vi "DSF.Shared.Configuration.Framework.Collapse Cluster.vi"(8 "error in (no error)":errorcluster, 11 "Framework Configuration in":refnum<class "DSF.Shared.Configuration.Framework.lvclass">) -> (0 "error out":errorcluster, 3 "Framework Configuration out":refnum<class "DSF.Shared.Configuration.Framework.lvclass">)   [LabVIEW 2017, in "DSF.Engine.lvlib" / "DSF.Shared.Configuration.Framework.lvclass"]
uses:
  DSF.Shared.Configuration.Framework.lvclass
  DSF.Shared.Configuration.Framework.lvclass/DSF.Shared.Configuration.Framework.ctl
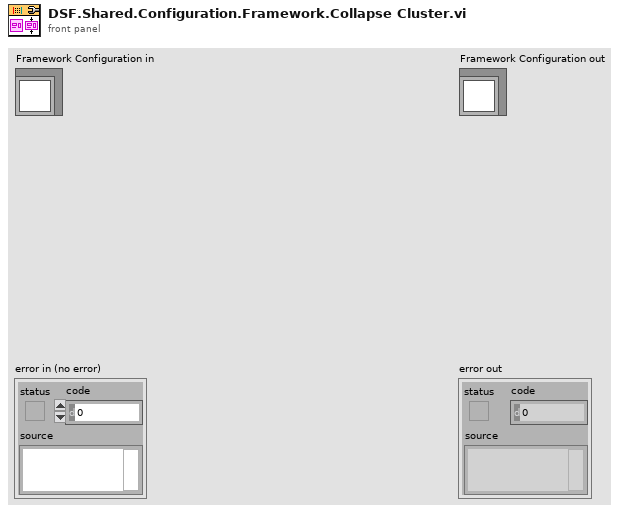
[diagram p1: front panel]
types:
  T1 = typedef "DSF.Engine.lvlib/DSF.Shared.Refactor.Typedefs.Framework Configuration.Aggregate.ctl" = cluster{"Plugins":T2[]}
  T2 = typedef "DSF.Engine.lvlib/DSF.Shared.Refactor.Typedefs.Plugin Configuration.Aggregate.ctl" = cluster{"name":string, "class":string, "cycle timing":T3, "Transfer Groups":T4[]}
  T3 = typedef "DSF.Engine.lvlib/DSF.Shared.Typedefs.Cycle Timing Factors.ctl" = cluster{"Priority":u64, "Decimation":u64, "Offset":u64}
  T4 = typedef "DSF.Engine.lvlib/DSF.Shared.Refactor.Typedefs.Transfer Group Configuration.Aggregate.ctl" = cluster{"name":string, "direction":T5, "cycle timing":T3, "Transfers":T6[]}
  T5 = typedef "DSF.Engine.lvlib/DSF.Shared.Typedefs.Direction.ctl" = enum8{"Tx", "Rx"}
  T6 = typedef "DSF.Engine.lvlib/DSF.Shared.Refactor.Typedefs.Transfer Configuration.ctl" = cluster{"name":string, "byte order":T7, "channel configurations":T8[]}
  T7 = typedef "DSF.Engine.lvlib/DSF.Shared.Typedefs.Byte Order.ctl" = enum8{"big-endian", "little-endian"}
  T8 = typedef "DSF.Engine.lvlib/DSF.Shared.Refactor.Typedefs.Channel Array Configuration.ctl" = cluster{"name":string, "data type":T9, "count":u64, "buffer offset":u64, "engine offset":u64}
  T9 = typedef "DSF.Engine.lvlib/DSF.Shared.Typedefs.Data Type.ctl" = enum8{"Bool", "SGL", "DBL", "I8", "I16", "I32", "I64", "U8", "U16", "U32", "U64"}
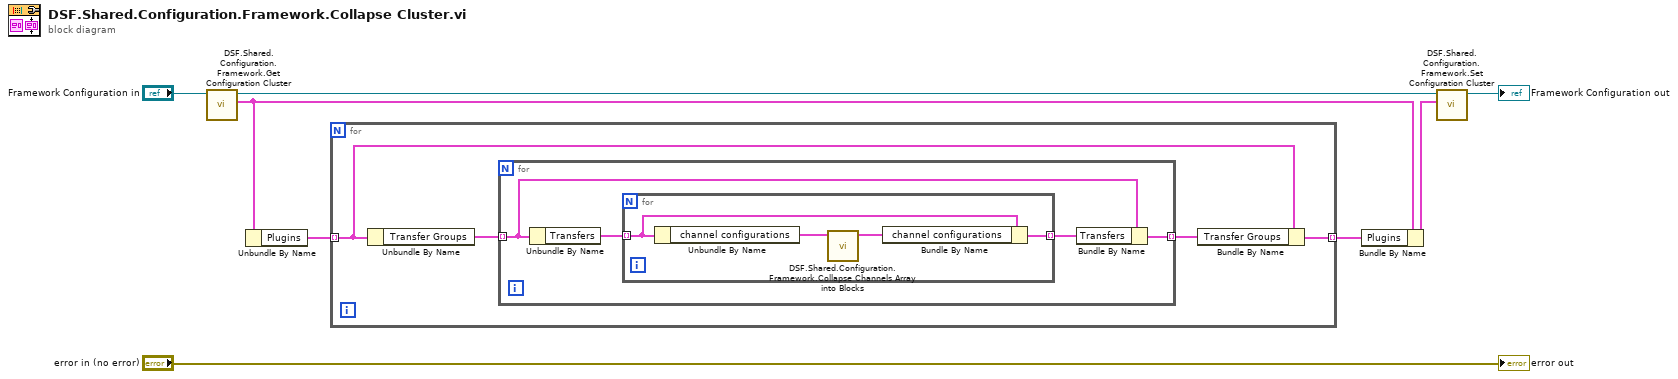
[diagram p0: block diagram]
diagram:
  n1 = call "DSF.Shared.Configuration.Framework.Get Configuration Cluster.vi"("Framework Configuration in"="Framework Configuration in") -> ("Framework Configuration"=w5:T1, "Framework Configuration out"=w7:refnum<class "DSF.Shared.Configuration.Framework.lvclass">)  [unwired: 9 in]
  n2 = Unbundle By Name(w5) -> ("Plugins"=w4:T2[])
  n3 = for {
    tunnel: w4 -> [w11] mode=indexing
    tunnel: [w9] -> w3 mode=indexing
    n4 = Unbundle By Name(w11) -> ("Transfer Groups"=w12:T4[])
    n5 = for {
      tunnel: w12 -> [w15] mode=indexing
      tunnel: [w13] -> w10 mode=indexing
      n6 = Unbundle By Name(w15) -> ("Transfers"=w16:T6[])
      n7 = for {
        tunnel: w16 -> [w19] mode=indexing
        tunnel: [w17] -> w14 mode=indexing
        n8 = Unbundle By Name(w19) -> ("channel configurations"=w20:T8[])
        n9 = call "DSF.Shared.Configuration.Framework.Collapse Channels Array into Blocks.vi"("channel configurations in"=w20) -> ("channel configurations out"=w18:T8[])  [unwired: 10 in]
        n10 = Bundle By Name(cluster=w19, "channel configurations"=w18) -> (w17:T6)
      }
      n11 = Bundle By Name(cluster=w15, "Transfers"=w14) -> (w13:T4)
    }
    n12 = Bundle By Name(cluster=w11, "Transfer Groups"=w10) -> (w9:T2)
  }
  n13 = Bundle By Name(cluster=w5, "Plugins"=w3) -> (w2:T1)
  n14 = call "DSF.Shared.Configuration.Framework.Set Configuration Cluster.vi"("Framework Configuration"=w2, "Framework Configuration in"=w7) -> ("Framework Configuration out"=→"Framework Configuration out":refnum<class "DSF.Shared.Configuration.Framework.lvclass">)  [unwired: 9 in]
  "error out" <- "error in (no error)"
